vi "GetTerms.vi"(0 "XRef":T12, 1 "State In":T10) -> (14 "Terms":T2, 15 "Fatal Error Out":T1)   [LabVIEW 2021, in "myRIO PWM Open.xnode"]
uses:
  <vilib>/myRIO/Instrument Drivers/Onboard IO/PWM/vis/myRIO PWM Open.xnode
  <vilib>/XNodeSupport/XNodeXNodeRef.ctl
  <vilib>/myRIO/Instrument Drivers/Onboard IO/PWM/vis/State.ctl
  <vilib>/myRIO/Common/Instrument Driver Framework/Utilities/typedefs/myRIOXPeripheral.ctl
  <vilib>/XNodeSupport/XNodeTerm4Array.ctl
  <vilib>/XNodeSupport/XNodeTerm4.ctl
  <vilib>/XNodeSupport/XNodeString.ctl
  <vilib>/XNodeSupport/XNodeVariant.ctl
  <vilib>/XNodeSupport/XNodeRect32.ctl
  <vilib>/XNodeSupport/XNodeInt.ctl
  <vilib>/XNodeSupport/XNodeBool.ctl
  <vilib>/XNodeSupport/XNodeTermDirection.ctl
  <vilib>/XNodeSupport/XNodeErrorCluster.ctl
  <vilib>/myRIO/Common/Instrument Driver Framework/Utilities/vis/myRIOXGlobal.vi
  <vilib>/XNodeSupport/NI_XNodeSupport.lvlib
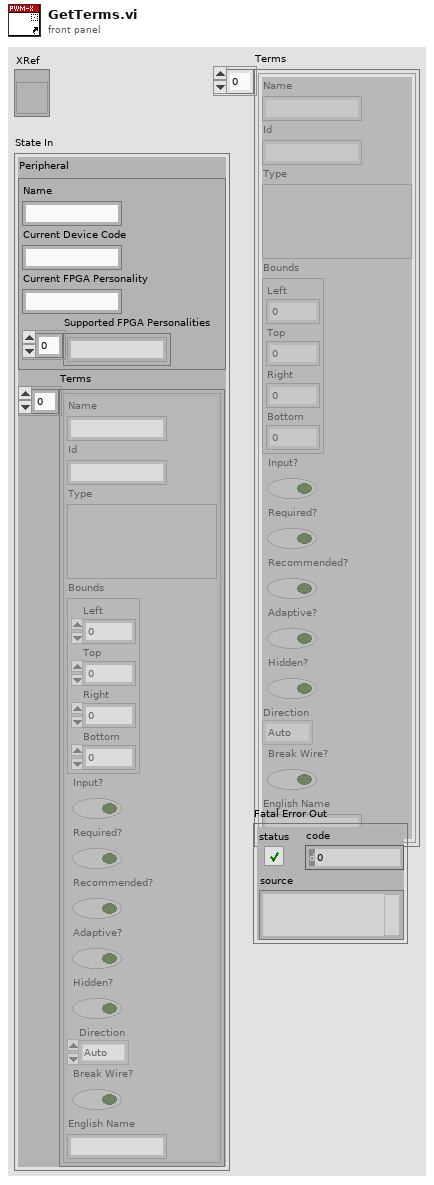
[diagram p1: front panel]
types:
  T1 = typedef "NI_XNodeSupport.lvlib/XNodeErrorCluster.ctl" = errorcluster
  T2 = typedef "NI_XNodeSupport.lvlib/XNodeTerm4Array.ctl" = T3[]
  T3 = typedef "NI_XNodeSupport.lvlib/XNodeTerm4.ctl" = cluster{"Name":T4, "Id":T4, "Type":T5, "Bounds":T6, "Input?":T8, "Required?":T8, "Recommended?":T8, "Adaptive?":T8, "Hidden?":T8, "Direction":T9, "Break Wire?":T8, "English Name":T4}
  T4 = typedef "NI_XNodeSupport.lvlib/XNodeString.ctl" = string
  T5 = typedef "NI_XNodeSupport.lvlib/XNodeVariant.ctl" = variant
  T6 = typedef "NI_XNodeSupport.lvlib/XNodeRect32.ctl" = cluster{"Left":T7, "Top":T7, "Right":T7, "Bottom":T7}
  T7 = typedef "NI_XNodeSupport.lvlib/XNodeInt.ctl" = i32
  T8 = typedef "NI_XNodeSupport.lvlib/XNodeBool.ctl" = bool
  T9 = typedef "NI_XNodeSupport.lvlib/XNodeTermDirection.ctl" = enum32{"Auto", "Up", "Down", "Left", "Right", "Center"}
  T10 = typedef "myRIO PWM Open.xnode/State.ctl" = cluster{"Peripheral":T11, "Terms":T2}
  T11 = typedef "myRIOXPeripheral.ctl" = cluster{"Name":string, "Current Device Code":string, "Current FPGA Personality":string, "Supported FPGA Personalities":string[]}
  T12 = typedef "NI_XNodeSupport.lvlib/XNodeXNodeRef.ctl" = refnum<vi>
  T13 = enum32{"Invalid Class", "File Path", "Variable", "Elemental IO", "VI Connector Pane", "VI Signature", "File No Warn", "Function Block Item", "Library Data", "Variable (Target Relative)", "Conditional Compile Symbol", "External Function"}
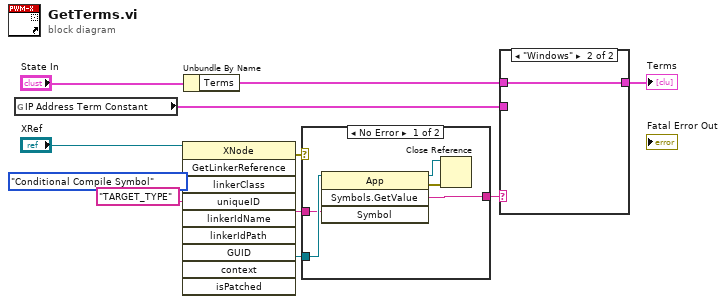
[diagram p0: block diagram]
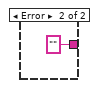
[diagram p2: hidden frame]
diagram:
  n1 = global read "myRIOXGlobal.vi" "IP Address Term Constant"() -> (w11:T3)
  n2 = invoke class="XNode" method="GetLinkerReference"(reference="XRef", "linkerClass"=T13."Conditional Compile Symbol", "uniqueID"="TARGET_TYPE") -> (error out=w1:errorcluster, "linkerIdName"=w4:string, "context"=w3:refnum<vi>)  [unwired: 7 in, 7 out]
  n3 = Unbundle By Name("State In") -> ("Terms"=w5:T2)
  n4 = case shown="No Error" w1 {
    tunnel: w3 -> [w16 _]
    tunnel: w4 -> [w15 _]
    tunnel: [w14 "" ("Symbols.GetValue")] -> w2
    frame No Error {
      n5 = invoke class="App" method="Symbols.GetValue"(reference=w16, "Symbol"=w15) -> (reference out=w12:refnum<vi>, error out=w13:errorcluster, "Symbols.GetValue"=w14:string)  [unwired: 2 in, 1 out]
      n6 = Close Reference(reference=w12, error in (no error)=w13) -> ()  [unwired: 1 out]
    }
    frame Error {
    }
  }
  n7 = case shown="\"Windows\"" w2 {
    tunnel: [w18 w19] -> w6
    tunnel: w11 -> [_ _]
    tunnel: w5 -> [w18 w19]
    frame "RT", Default {
    }
    frame "Windows" {
    }
  }
  "Terms" <- w6
